vi "Teleop.vi"   [LabVIEW 2016]
doc: "This VI is called for each TeleOp packet received from the DS where the robot is not disabled. It is often used to read from the joysticks and update I/O or to update setpoints for timed control loops. It should complete and return within 20 milliseconds or it may miss DS packets."
uses:
  <vilib>/Rock Robotics/WPI/Utilities/WPI_GetSetVariantRefNum.vi
  External/2ndContollerStatus.vi
  External/External.lvlib
types:
  T1 = enum16{"A", "B", "X", "Y", "LB", "RB", "Back", "Start", "Left Joystick Pressure Button", "Right Joystick Pressure Button"}
  T2 = enum16{"Left X Axis", "Left Y Axis", "Left Trigger", "Right Trigger", "Right X Axis", "Right Y Axis"}
  T3 = typedef "WPI_JoystickDevRef.ctl" = cluster{"Device":T4}
  T4 = typedef "WPI_JoystickDeviceEnum.ctl" = enum16{"USB 0", "USB 1", "USB 2", "USB 3", "USB 4", "USB 5"}
  T5 = typedef "WPI_RobotDriveDevRef.ctl" = cluster{"DevStatus":errorcluster, "Motors[]":T6[], "Square Inputs":bool, "Max Output":dbl}
  T6 = typedef "WPI_MotorControlDeviceRef.ctl" = cluster{"DeviceStatus":errorcluster, "Type":T7, "PWM":cluster{"PWM Channel":T8, "DeadBand":T9}, "CAN":cluster{"Device Number":u8, "SetOutput VI Ref":variant, "GetOutput VI Ref":variant, "Enable VI Ref":variant, "Disable VI Ref":variant, "Data":variant}, "Invert":bool}
  T7 = typedef "WPI_MotorControlType.ctl" = enum16{"PWM", "CAN"}
  T8 = typedef "FPGA_DIOPWMChannel.ctl" = enum8{"PWM 0", "PWM 1", "PWM 2", "PWM 3", "PWM 4", "PWM 5", "PWM 6", "PWM 7", "PWM 8", "PWM 9", "PWM MXP 0", "PWM MXP 1", "PWM MXP 2", "PWM MXP 3", "PWM MXP 4", "PWM MXP 5", "PWM MXP 6", "PWM MXP 7", "PWM MXP 8", "PWM MXP 9", "Invalid"}
  T9 = typedef "WPI_PWMDeadband.ctl" = cluster{"Name":string, "maxPositivePwm":i32, "minPositivePwm":i32, "centerPwm":i32, "maxNegativePwm":i32, "minNegativePwm":i32, "angularRange":u16}
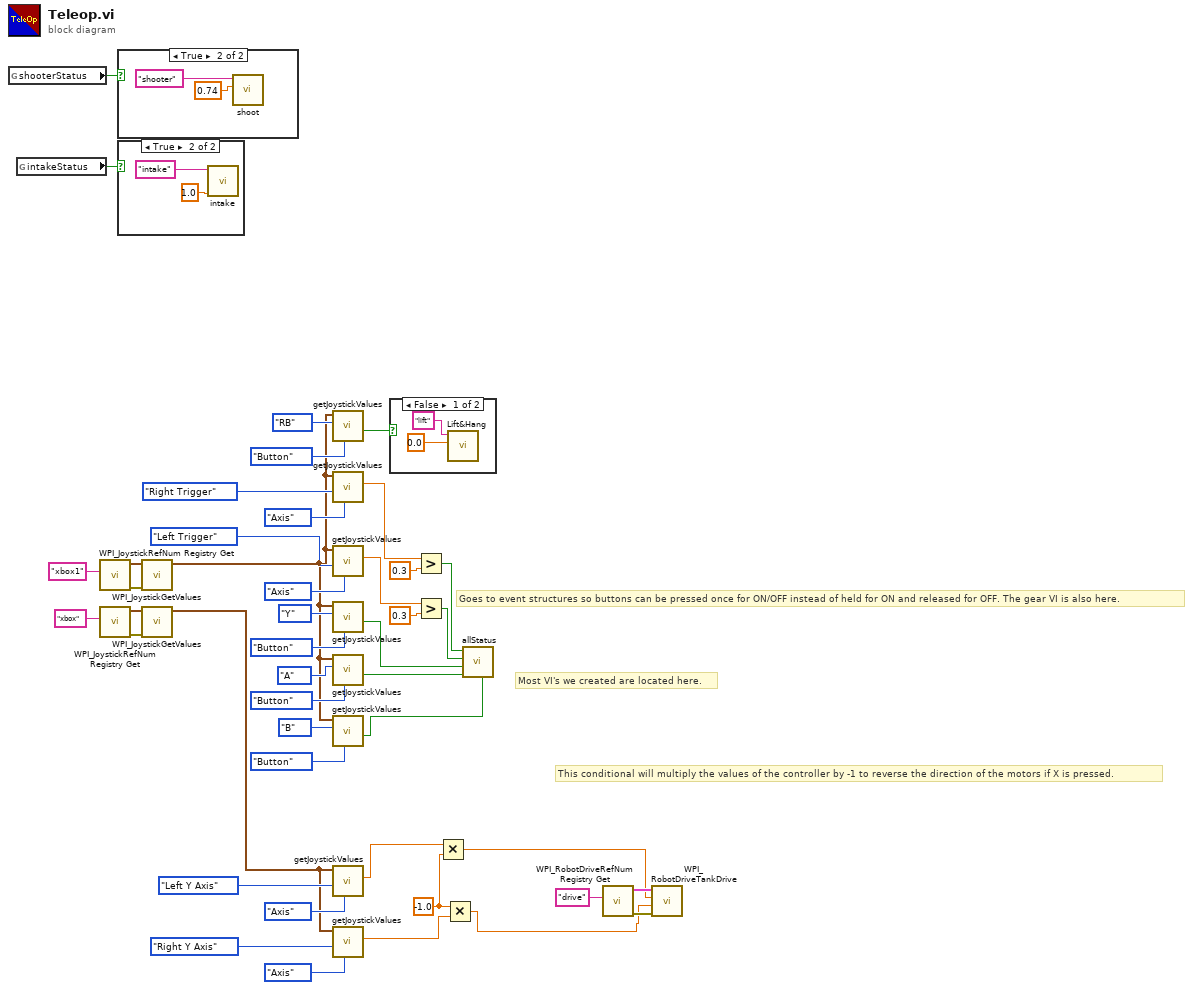
[diagram p0: block diagram]
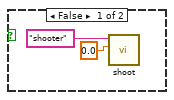
[diagram p2: hidden frame]
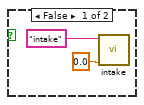
[diagram p3: hidden frame]
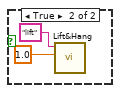
[diagram p4: hidden frame]
diagram:
  w5 = -1.0 ("x")
  # "Most VI's we created are located here."
  # "This conditional will multiply the values of the controller by -1 to reverse the direction of the motors if X is pressed."
  # "Goes to event structures so buttons can be pressed once for ON/OFF instead of held for ON and released for OFF. The gear VI is also here."
  n1 = global read "2ndContollerStatus.vi" "shooterStatus"() -> (w35:bool)
  n2 = global read "2ndContollerStatus.vi" "intakeStatus"() -> (w36:bool)
  n3 = call <vilib>:"WPI_JoystickRefNum Registry Get.vi"("refnum name"="xbox1") -> ("error out"=w9:errorcluster, "JoystickDevRef"=w8:T3)  [unwired: 9 in]
  n4 = call <vilib>:"WPI_JoystickRefNum Registry Get.vi"("refnum name"="xbox") -> ("error out"=w12:errorcluster, "JoystickDevRef"=w11:T3)  [unwired: 9 in]
  n5 = case shown="True" w35 {
    frame False {
      n6 = call "shoot.vi"("Motor Power"=0.0, "refnum name"="shooter") -> ()  [unwired: 9 in, 1 out]
    }
    frame True {
      n7 = call "shoot.vi"("Motor Power"=0.74, "refnum name"="shooter") -> ()  [unwired: 9 in, 1 out]
    }
  }
  n8 = case shown="True" w36 {
    frame False {
      n9 = call "intake.vi"("intakeSpeed"=0.0, "intake"="intake") -> ()  [unwired: 9 in, 1 out]
    }
    frame True {
      n10 = call "intake.vi"("intakeSpeed"=1.0, "intake"="intake") -> ()  [unwired: 9 in, 1 out]
    }
  }
  n11 = call <vilib>:"WPI_JoystickGetValues.vi"("error in (no error)"=w9, "JoystickDevRef"=w8) -> ("JoystickDevRef"=w7:T3)  [unwired: 5 in, 4 out]
  n12 = call <vilib>:"WPI_JoystickGetValues.vi"("error in (no error)"=w12, "JoystickDevRef"=w11) -> ("JoystickDevRef"=w6:T3)  [unwired: 5 in, 4 out]
  n13 = call "getJoystickValues.vi"("Mode"=enum16{"Axis", "Button", "POV"}."Button", "buttonType"=T1."RB", "JoystickDevRef"=w7) -> ("Button Pressed"=w44:bool)  [unwired: 5 in, 3 out]
  n14 = call "getJoystickValues.vi"("Mode"=enum16{"Axis", "Button", "POV"}."Axis", "axisType"=T2."Right Trigger", "JoystickDevRef"=w7) -> ("Value"=w38:dbl)  [unwired: 5 in, 3 out]
  n15 = call "getJoystickValues.vi"("Mode"=enum16{"Axis", "Button", "POV"}."Axis", "axisType"=T2."Left Trigger", "JoystickDevRef"=w7) -> ("Value"=w37:dbl)  [unwired: 5 in, 3 out]
  n16 = call "getJoystickValues.vi"("Mode"=enum16{"Axis", "Button", "POV"}."Button", "buttonType"=T1."Y", "JoystickDevRef"=w7) -> ("Button Pressed"=w30:bool)  [unwired: 5 in, 3 out]
  n17 = call "getJoystickValues.vi"("Mode"=enum16{"Axis", "Button", "POV"}."Button", "buttonType"=T1."A", "JoystickDevRef"=w7) -> ("Button Pressed"=w32:bool)  [unwired: 5 in, 3 out]
  n18 = call "getJoystickValues.vi"("Mode"=enum16{"Axis", "Button", "POV"}."Button", "buttonType"=T1."B", "JoystickDevRef"=w7) -> ("Button Pressed"=w31:bool)  [unwired: 5 in, 3 out]
  n19 = call "getJoystickValues.vi"("Mode"=enum16{"Axis", "Button", "POV"}."Axis", "axisType"=T2."Left Y Axis", "JoystickDevRef"=w6) -> ("Value"=w4:dbl)  [unwired: 5 in, 3 out]
  n20 = call "getJoystickValues.vi"("Mode"=enum16{"Axis", "Button", "POV"}."Axis", "axisType"=T2."Right Y Axis", "JoystickDevRef"=w6) -> ("Value"=w2:dbl)  [unwired: 5 in, 3 out]
  n21 = case shown="False" w44 {
    frame False {
      n22 = call "Lift&Hang.vi"("status"=0.0, "refnum name"="lift" ("lift")) -> ()  [unwired: 9 in, 1 out]
    }
    frame True {
      n23 = call "Lift&Hang.vi"("status"=1.0, "refnum name"="lift" ("lift")) -> ()  [unwired: 9 in, 1 out]
    }
  }
  n24 = Greater?(x=w38, y=0.3) -> (0:w34:bool)
  n25 = Greater?(x=w37, y=0.3) -> (0:w33:bool)
  n26 = Multiply(x=w4, y=w5) -> (x*y=w3:dbl)
  n27 = Multiply(x=w5, y=w2) -> (x*y=w1:dbl)
  n28 = call "allStatus.vi"("intake"=w31, "gear"=w32, "shooter"=w30, "hopper1"=w33, "hopper0"=w34) -> ()  [unwired: 7 in]
  n29 = call <vilib>:"WPI_RobotDriveRefNum Registry Get.vi"("refnum name"="drive") -> ("error out"=w42:errorcluster, "RobotDriveDevRef"=w43:T5)  [unwired: 9 in]
  n30 = call <vilib>:"WPI_RobotDriveTankDrive.vi"("error in (no error)"=w42, "Right axis value"=w1, "Left axis value"=w3, "RobotDriveDevRef"=w43) -> ()  [unwired: 5 in, 3 out]
